vi "Helper - InterpretKeyPress.vi"(4 "Sail Key Control Config":T4={"Sail Position Max"=1.0, "Sail Position Increment"=0.025}, 6 "Rudder Key Control Config":T2={"Rudder Angle Max"=50.0, "Rudder Angle Increment"=5.0}, 8 "FocusObj":refnum<vi>, 9 "VKey":T1=enum."Up", 10 "Char":i16, 11 "Command In":T6={"Sail Position"=0.0, "Rudder Angle"=6.0}) -> (3 "Command Out":T6={"Sail Position"=0.0, "Rudder Angle"=6.0})   [LabVIEW 2011]
doc: "Update sailboat commands (rudder angle and sail position currently) according to key presses. Configuration options are exposed which allow the upper range of the value to be selected and the increment associated with the appropriate key press.\n\nThe FocusObj input should come from the appropriate event structure event. When no particular control or indicator has the focus, the key presses will update the command input.\n\nAssumptions:\n- the minimum value for all commands is 0\n\nAuthor: Jared Kirschner"
uses:
  2-Think/2 Typedefs/setpoints to boat.ctl
  2-Think/2 Typedefs/sail setpt.ctl
  2-Think/2 Typedefs/rudder angle.ctl
  0 Typedefs/sailKeyControlConfig.ctl
  0 Typedefs/rudderKeyControlConfig.ctl
  <vilib>/event_ctls.llb/eventvkey.ctl
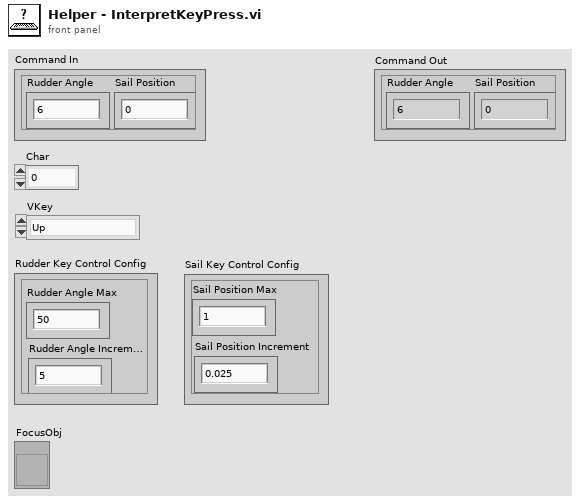
[diagram p1: front panel]
types:
  T1 = typedef "eventvkey.ctl" = enum16{"ASCII", "Enter", "Return", "Shift", "Ctrl", "Alt", "Cmd", "Opt", "Caps", "NumLock", "Clear", "Break", "Up", "Down", "Left", "Right", "Insert", "Delete", "Home", "End", "PageUp", "PageDown", "Escape", "Help", "Pause", "ScrollLock", "F1", "F2", "F3", "F4", "F5", "F6", "F7", "F8", "F9", "F10", "F11", "F12", "F13", "F14", "F15", "F16", "F17", "F18", "F19", "F20", "F21", "F22", "F23", "F24", "Play", "VolumeUp", "VolumeDown", "Mute", "Two Byte Char"}
  T2 = typedef "rudderKeyControlConfig.ctl" = cluster{"Rudder Angle Max":T3, "Rudder Angle Increment":T3}
  T3 = typedef "rudder angle.ctl" = dbl
  T4 = typedef "sailKeyControlConfig.ctl" = cluster{"Sail Position Max":T5, "Sail Position Increment":T5}
  T5 = typedef "sail setpt.ctl" = dbl
  T6 = typedef "setpoints to boat.ctl" = cluster{"Sail Position":T5, "Rudder Angle":T3}
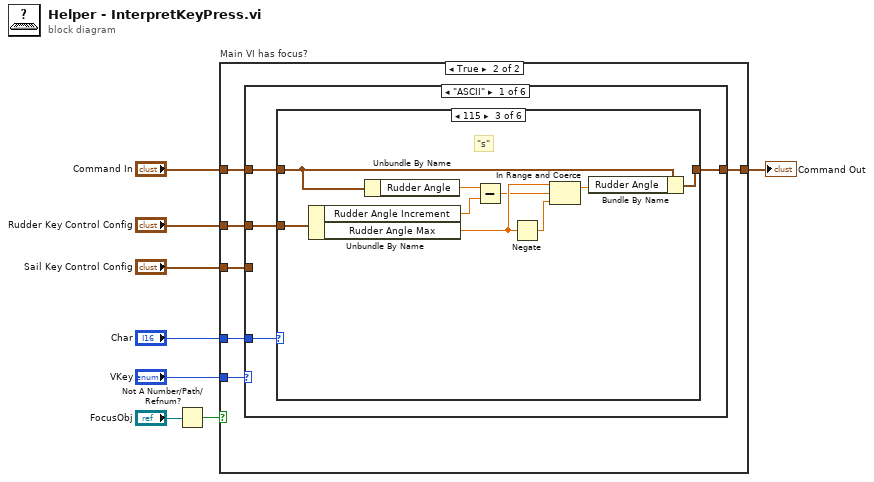
[diagram p0: block diagram]
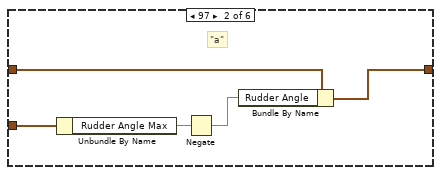
[diagram p4: hidden frame]
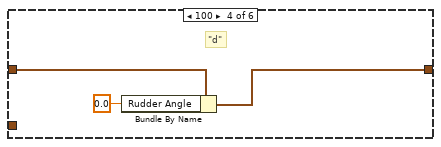
[diagram p5: hidden frame]
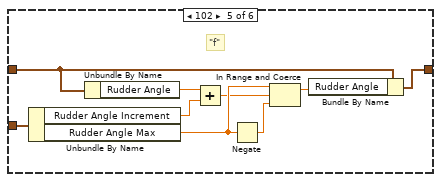
[diagram p6: hidden frame]
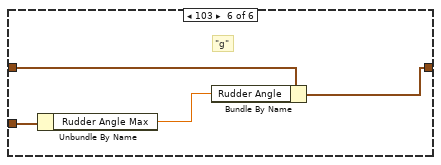
[diagram p7: hidden frame]
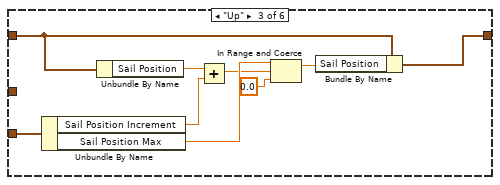
[diagram p9: hidden frame]
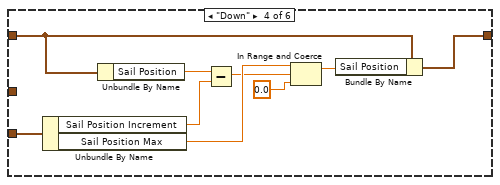
[diagram p10: hidden frame]
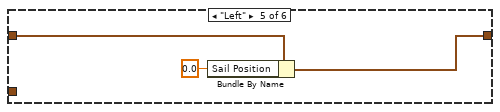
[diagram p11: hidden frame]
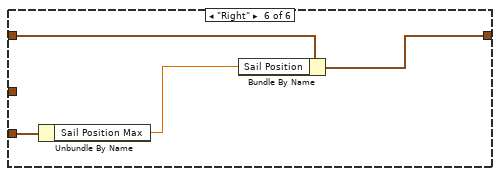
[diagram p12: hidden frame]
diagram:
  n1 = Not A Number/Path/Refnum?(number/path/refnum="FocusObj") -> (NaN/Path/Refnum?=w1:bool)
  n2 = case "Main VI has focus?" shown="True" w1 {
    tunnel: "VKey" -> [_ w15]
    tunnel: "Command In" -> [w9 w14]
    tunnel: "Rudder Key Control Config" -> [_ w13]
    tunnel: "Sail Key Control Config" -> [_ w12]
    tunnel: "Char" -> [_ w11]
    tunnel: [w9 w10] -> w3
    frame False {
    }
    frame True {
      n3 = case shown="\"ASCII\"" w15 {
        tunnel: w14 -> [w18 w51 w53 w63 w71 w74]
        tunnel: w13 -> [w16 _ _ _ _ _]
        tunnel: w12 -> [_ _ w54 w62 _ w75]
        tunnel: w11 -> [w19 _ _ _ _ _]
        tunnel: [w17 w51 w52 w61 w70 w73] -> w10
        frame "ASCII" {
          n4 = case shown="115" w19 {
            tunnel: w18 -> [w20 w23 w27 w36 w39 w48]
            tunnel: [w20 w22 w26 w35 w38 w47] -> w17
            tunnel: w16 -> [_ w21 w28 _ w40 w49]
            frame 0, Default {
            }
            frame 97 {
              # "\"a\""
              n5 = Unbundle By Name(w21) -> ("Rudder Angle Max"=w24:T3)
              n6 = Negate(x=w24) -> (-x=w25:T3)
              n7 = Bundle By Name(cluster=w23, "Rudder Angle"=w25) -> (w22:T6)
            }
            frame 115 {
              # "\"s\""
              n8 = Unbundle By Name(w28) -> ("Rudder Angle Increment"=w31:T3, "Rudder Angle Max"=w33:T3)
              n9 = Unbundle By Name(w27) -> ("Rudder Angle"=w29:T3)
              n10 = Subtract(x=w29, y=w31) -> (x-y=w30:T3)
              n11 = Negate(x=w33) -> (-x=w32:T3)
              n12 = In Range and Coerce(upper limit=w33, x=w30, lower limit=w32) -> (coerced(x)=w34:T3)  [unwired: 1 out]
              n13 = Bundle By Name(cluster=w27, "Rudder Angle"=w34) -> (w26:T6)
            }
            frame 100 {
              # "\"d\""
              n14 = Bundle By Name(cluster=w36, "Rudder Angle"=T3 0.0) -> (w35:T6)
            }
            frame 102 {
              # "\"f\""
              n15 = Unbundle By Name(w40) -> ("Rudder Angle Increment"=w43:T3, "Rudder Angle Max"=w45:T3)
              n16 = Unbundle By Name(w39) -> ("Rudder Angle"=w41:T3)
              n17 = Add(x=w41, y=w43) -> (x+y=w42:T3)
              n18 = Negate(x=w45) -> (-x=w44:T3)
              n19 = In Range and Coerce(upper limit=w45, x=w42, lower limit=w44) -> (coerced(x)=w46:T3)  [unwired: 1 out]
              n20 = Bundle By Name(cluster=w39, "Rudder Angle"=w46) -> (w38:T6)
            }
            frame 103 {
              # "\"g\""
              n21 = Unbundle By Name(w49) -> ("Rudder Angle Max"=w50:T3)
              n22 = Bundle By Name(cluster=w48, "Rudder Angle"=w50) -> (w47:T6)
            }
          }
        }
        frame Default {
        }
        frame "Up" {
          n23 = Unbundle By Name(w54) -> ("Sail Position Increment"=w56:T5, "Sail Position Max"=w58:T5)
          n24 = Unbundle By Name(w53) -> ("Sail Position"=w55:T5)
          n25 = Add(x=w55, y=w56) -> (x+y=w57:T5)
          n26 = In Range and Coerce(upper limit=w58, x=w57, lower limit=T5 0.0 ("Sail Position")) -> (coerced(x)=w60:T5)  [unwired: 1 out]
          n27 = Bundle By Name(cluster=w53, "Sail Position"=w60) -> (w52:T6)
        }
        frame "Down" {
          n28 = Unbundle By Name(w62) -> ("Sail Position Increment"=w65:T5, "Sail Position Max"=w67:T5)
          n29 = Unbundle By Name(w63) -> ("Sail Position"=w64:T5)
          n30 = Subtract(x=w64, y=w65) -> (x-y=w66:T5)
          n31 = In Range and Coerce(upper limit=w67, x=w66, lower limit=T5 0.0 ("Sail Position")) -> (coerced(x)=w69:T5)  [unwired: 1 out]
          n32 = Bundle By Name(cluster=w63, "Sail Position"=w69) -> (w61:T6)
        }
        frame "Left" {
          n33 = Bundle By Name(cluster=w71, "Sail Position"=T5 0.0) -> (w70:T6)
        }
        frame "Right" {
          n34 = Unbundle By Name(w75) -> ("Sail Position Max"=w76:T5)
          n35 = Bundle By Name(cluster=w74, "Sail Position"=w76) -> (w73:T6)
        }
      }
    }
  }
  "Command Out" <- w3
